vi "Write ProductInfo.vi"(8 "error in (no error)":errorcluster, 10 "ProductInfo":string, 11 "GeneralCar in":refnum<class "GeneralCar.lvclass">) -> (0 "error out":errorcluster, 3 "GeneralCar out":refnum<class "GeneralCar.lvclass">)   [LabVIEW 2021, in "GeneralCar.lvclass"]
uses:
  GeneralCar.lvclass
  GeneralCar.lvclass/GeneralCar.ctl
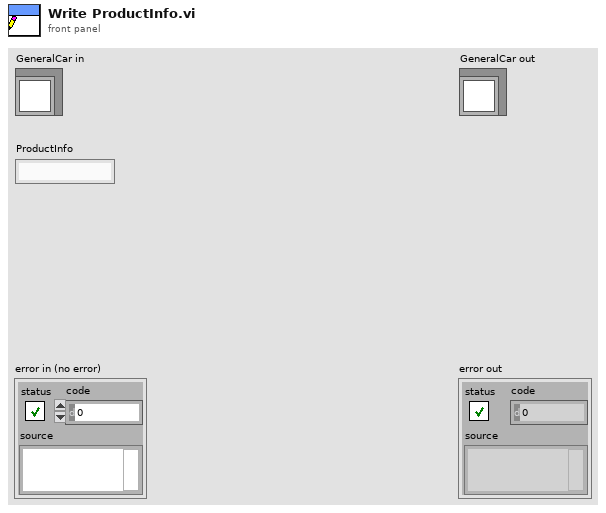
[diagram p1: front panel]
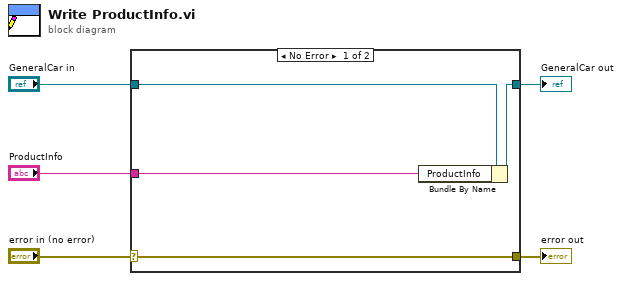
[diagram p0: block diagram]
diagram:
  n1 = case shown="No Error" "error in (no error)" {
    selector: "error in (no error)" -> [w9 w10]
    tunnel: [w9 w10] -> w4
    tunnel: [w7 w11] -> w2
    tunnel: "GeneralCar in" -> [w8 w11]
    tunnel: "ProductInfo" -> [w6 _]
    frame No Error {
      n2 = Bundle By Name(cluster=w8, "ProductInfo"=w6) -> (w7:refnum<class "GeneralCar.lvclass">)
    }
    frame Error {
    }
  }
  "error out" <- w4
  "GeneralCar out" <- w2
